vi "DSF.Engine.Status.Framework.Set Performance.vi"(10 "Framework Performance":refnum<class "DSF.Engine.Status.Framework.Performance.lvclass">, 11 "Framework Status in":refnum<class "DSF.Engine.Status.Framework.lvclass">) -> (3 "Framework Status out":refnum<class "DSF.Engine.Status.Framework.lvclass">)   [LabVIEW 2017, in "DSF.Engine.lvlib" / "DSF.Engine.Status.Framework.lvclass"]
uses:
  DSF.Engine.Status.Framework.lvclass
  DSF.Engine.Status.Framework.Performance.lvclass
  DSF.Engine.Status.Framework.lvclass/DSF.Engine.Status.Framework.ctl
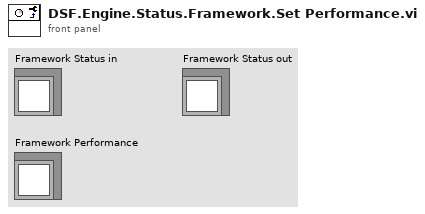
[diagram p1: front panel]
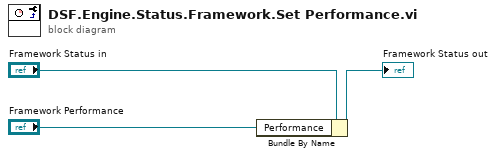
[diagram p0: block diagram]
diagram:
  n1 = Bundle By Name(cluster="Framework Status in", "Performance"="Framework Performance") -> (→"Framework Status out":refnum<class "DSF.Engine.Status.Framework.lvclass">)
